vi "MGI Running Average(DBL[][]).vi"(5 "Averaging Size":i32, 6 "Average Type(FIR)":T1, 7 "Initialize? (F)":bool, 11 "Value[chan][samp]":dbl[][](array[numeric])) -> (3 "Average[chan]":dbl[](array[numeric]))   [LabVIEW 2016]
doc: "Keep running averages of each of the input values. Infinite Impulse Response requires less processing, but it takes infinite time to arrive at a steady state value. Finite Impulse Reponse maintains an array of the specified size but is able to output means.\nThis VI is a reentrant functional global.\n\nAuthored by Shawn Walpole\nsupport@mooregoodideas.com\nwww.mooregoodideas.com\n\nCopyright (c) 2010, Moore Good Ideas, Inc.\n\nAll rights reserved.\n\nRedistribution and use in source and binary forms, with or without modification, are permitted provided that the following conditions are met:\n\n * Redistributions of source code must retain the above copyright notice, this list of conditions and the following disclaimer.\n * Redistributions in binary form must reproduce the above copyright notice, this list of conditions and the following disclaimer in the documentation and/or other materials provided with the distribution.\n * Neither the name of Moore Good Ideas, Inc. nor the names of its contributors may be used to endorse or promote products derived from this software without specific prior written permission.\n\nTHIS SOFTWARE IS PROVIDED BY THE COPYRIGHT HOLDERS AND CONTRIBUTORS \"AS IS\" AND ANY EXPRESS OR IMPLIED WARRANTIES, INCLUDING, BUT NOT LIMITED TO, THE IMPLIED WARRANTIES OF MERCHANTABILITY AND FITNESS FOR A PARTICULAR PURPOSE ARE DISCLAIMED. IN NO EVENT SHALL THE COPYRIGHT OWNER OR CONTRIBUTORS BE LIABLE FOR ANY DIRECT, INDIRECT, INCIDENTAL, SPECIAL, EXEMPLARY, OR CONSEQUENTIAL DAMAGES (INCLUDING, BUT NOT LIMITED TO, PROCUREMENT OF SUBSTITUTE GOODS OR SERVICES; LOSS OF USE, DATA, OR PROFITS; OR BUSINESS INTERRUPTION) HOWEVER CAUSED AND ON ANY THEORY OF LIABILITY, WHETHER IN CONTRACT, STRICT LIABILITY, OR TORT (INCLUDING NEGLIGENCE OR OTHERWISE) ARISING IN ANY WAY OUT OF THE USE OF THIS SOFTWARE, EVEN IF ADVISED OF THE POSSIBILITY OF SUCH DAMAGE."
uses:
  <userlib>/_MGI/1D Array/MGI Average Type Enum.ctl
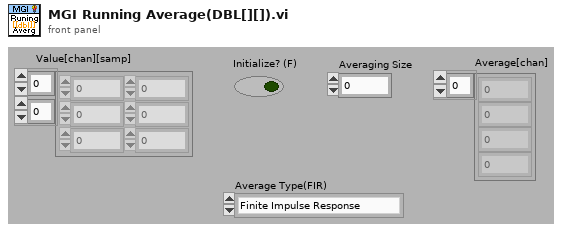
[diagram p1: front panel]
types:
  T1 = typedef "MGI Average Type Enum.ctl" = enum16{"Finite Impulse Response", "Infinite Impulse Response"}
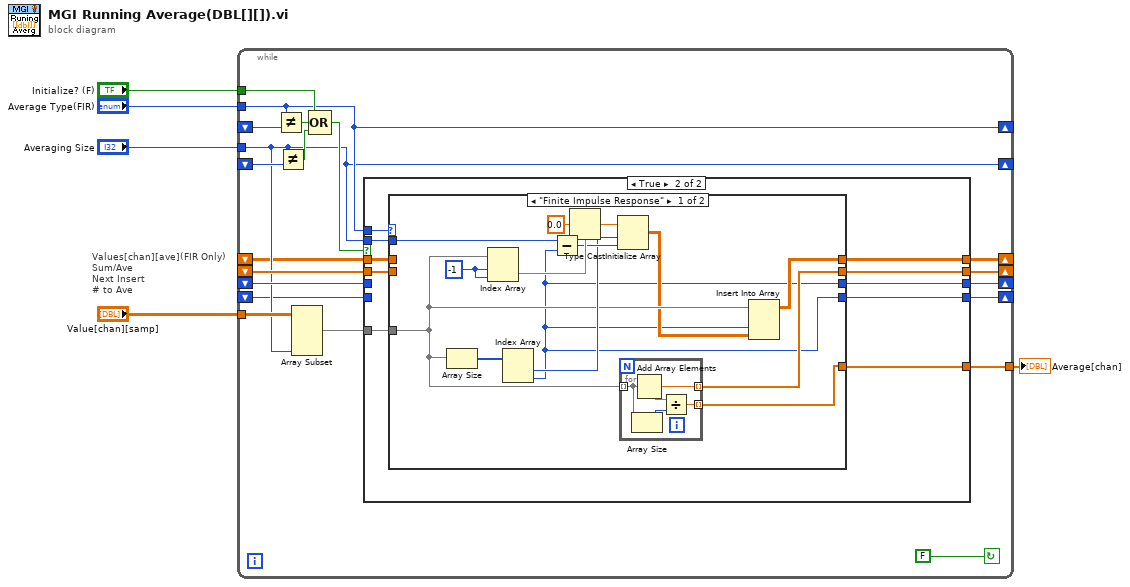
[diagram p0: block diagram]
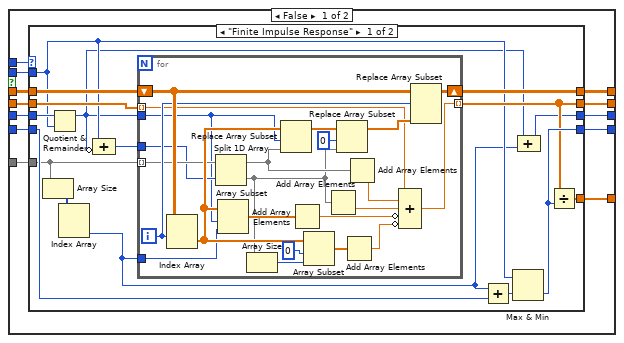
[diagram p2: hidden frame]
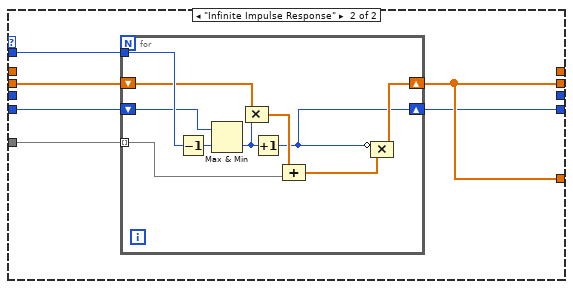
[diagram p3: hidden frame]
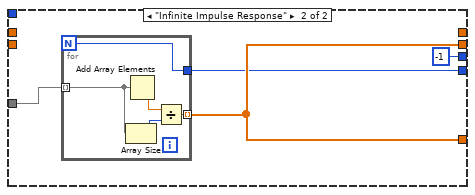
[diagram p4: hidden frame]
diagram:
  # "Values[chan][ave](FIR Only)\nSum/Ave\nNext Insert\n# to Ave"
  n1 = while {
    tunnel: "Averaging Size" -> [w9]
    tunnel: "Value[chan][samp]" -> [w11]
    shift-left: _ -> [w18]
    shift-right: [w20] -> _
    tunnel: "Initialize? (F)" -> [w23]
    shift-left: _ -> [w6]
    shift-right: [w17] -> _
    tunnel: "Average Type(FIR)" -> [w15]
    shift-right: [w15] -> _
    shift-left: _ -> [w24]
    shift-right: [w21] -> _
    shift-left: _ -> [w19]
    shift-right: [w9] -> _
    shift-left: _ -> [w22]
    tunnel: [w16] -> w2
    shift-right: [w8] -> _
    shift-left: _ -> [w7]
    stop <- FALSE continue-if-true
    n2 = Not Equal?(x=w15, y=w24) -> (x != y?=w14:bool)
    n3 = Not Equal?(x=w9, y=w22) -> (x != y?=w12:bool)
    n4 = Array Subset(array=w11, length (col)=w9) -> (w10:dbl[][])  [unwired: 3 in]
    n5 = Compound Arithmetic op=OR(w23, w14, w12) -> (w13:bool)
    n6 = case shown="True" w13 {
      tunnel: [w31 w94] -> w21
      tunnel: w10 -> [w33 w97]
      tunnel: [w29 w96] -> w20
      tunnel: w19 -> [w36 _]
      tunnel: w18 -> [w35 w100]
      tunnel: w6 -> [w34 w98]
      tunnel: w9 -> [w32 w101]
      tunnel: w15 -> [w37 w102]
      tunnel: [w30 w99] -> w17
      tunnel: [w28 w95] -> w16
      tunnel: [w26 w93] -> w8
      tunnel: w7 -> [w27 _]
      frame False {
        n7 = case shown="\"Finite Impulse Response\"" w37 {
          tunnel: w36 -> [w43 _]
          tunnel: w35 -> [w52 w81]
          tunnel: w34 -> [w53 _]
          tunnel: w33 -> [w45 w80]
          tunnel: w32 -> [w42 w82]
          tunnel: [w39 _] -> w31
          tunnel: [w51 _] -> w30
          tunnel: [w47 w78] -> w29
          tunnel: [w50 w78] -> w28
          tunnel: w27 -> [w46 w79]
          tunnel: [w48 w77] -> w26
          frame "Finite Impulse Response" {
            n8 = Array Size(array=w45) -> (size(s)=w44:i32[])
            n9 = Quotient & Remainder(x=w43, y=w42) -> (x-y*floor(x/y)=w40:i32)  [unwired: 1 out]
            n10 = Index Array(array=w44) -> (element #2=w38:i32)  [unwired: 2 in, 1 out]
            n11 = Compound Arithmetic op=ADD(w42, invert w40) -> (w41:i32)
            n12 = for {
              tunnel: w45 -> [w61] mode=indexing
              shift-right: [w75] -> w51
              shift-left: w53 -> [w76]
              tunnel: w52 -> [w70] mode=indexing
              tunnel: [w68] -> w47 mode=indexing
              tunnel: w38 -> [w54]
              tunnel: w41 -> [w60]
              tunnel: w40 -> [w55]
              i -> [w74]
              n13 = Index Array(array=w76, index (row)=w74) -> (element=w73:dbl[])  [unwired: 1 in]
              n14 = Split 1D Array(array=w61, index=w60) -> (first subarray=w59:dbl[], second subarray=w57:dbl[])
              n15 = Array Subset(array=w73, index=w55, length=w54) -> (w67:dbl[])
              n16 = Array Size(array=w57) -> (size(s)=w56:i32)
              n17 = Replace Array Subset(array=w73, new element=w59, index=w55) -> (w72:dbl[])
              n18 = Add Array Elements(numeric array=w67) -> (sum=w66:dbl)
              n19 = Array Subset(array=w73, index=0, length=w56) -> (w69:dbl[])
              n20 = Add Array Elements(numeric array=w57) -> (sum=w64:dbl)
              n21 = Replace Array Subset(array=w72, new element=w57, index=0) -> (w71:dbl[])
              n22 = Add Array Elements(numeric array=w69) -> (sum=w65:dbl)
              n23 = Add Array Elements(numeric array=w59) -> (sum=w63:dbl)
              n24 = Compound Arithmetic op=ADD(w70, w63, w64, invert w66, invert w65) -> (w68:dbl)
              n25 = Replace Array Subset(array=w76, new element=w71, index (row)=w74) -> (w75:dbl[][])  [unwired: 1 in]
            }
            n26 = Add(x=w38, y=w46) -> (x+y=w49:i32)
            n27 = Max & Min(x=w42, y=w49) -> (min(x,y)=w48:i32)  [unwired: 1 out]
            n28 = Compound Arithmetic op=ADD(w40, w38) -> (w39:i32)
            n29 = Divide(x=w47, y=w48) -> (x/y=w50:dbl[])
          }
          frame "Infinite Impulse Response" {
            n30 = for {
              tunnel: w82 -> [w92]
              tunnel: w80 -> [w89] mode=indexing
              shift-right: [w85] -> w78
              shift-left: w81 -> [w90]
              shift-right: [w83] -> w77
              shift-left: w79 -> [w84]
              n31 = Decrement(x=w92) -> (x-1=w91:i32)
              n32 = Max & Min(x=w84, y=w91) -> (min(x,y)=w86:i32)  [unwired: 1 out]
              n33 = Compound Arithmetic op=MULTIPLY(w90, w86) -> (w88:dbl[])
              n34 = Increment(x=w86) -> (x+1=w83:i32)
              n35 = Compound Arithmetic op=ADD(w88, w89) -> (w87:dbl[])
              n36 = Compound Arithmetic op=MULTIPLY(invert w83, w87) -> (w85:dbl[])
            }
          }
        }
      }
      frame True {
        n37 = case shown="\"Finite Impulse Response\"" w102 {
          tunnel: w101 -> [w111 _]
          tunnel: w100 -> [_ _]
          tunnel: [w105 _] -> w99
          tunnel: w98 -> [_ _]
          tunnel: w97 -> [w106 w123]
          tunnel: [w110 w124] -> w96
          tunnel: [w109 w124] -> w95
          tunnel: [w103 -1] -> w94
          tunnel: [w103 w121] -> w93
          frame "Finite Impulse Response" {
            w115 = -1 ("index (row)")
            n38 = Array Size(array=w106) -> (size(s)=w112:i32[])
            n39 = Index Array(array=w106, index (row)=w115, index (col)=w115) -> (element=w114:dbl)
            n40 = Index Array(array=w112) -> (element #1=w107:i32, element #2=w103:i32)  [unwired: 2 in]
            n41 = Subtract(x=w111, y=w103) -> (x-y=w108:i32)
            n42 = Type Cast(type=w114, x=0.0 ("element")) -> (*(type *) &x=w113:dbl)
            n43 = Initialize Array(w113, w107, w108) -> (w104:dbl[][])
            n44 = for {
              tunnel: w106 -> [w119] mode=indexing
              tunnel: [w120] -> w110 mode=indexing
              tunnel: [w117] -> w109 mode=indexing
              n45 = Array Size(array=w119) -> (size(s)=w118:i32)
              n46 = Add Array Elements(numeric array=w119) -> (sum=w120:dbl)
              n47 = Divide(x=w120, y=w118) -> (x/y=w117:dbl)
            }
            n48 = Insert Into Array(array=w106, index (col)=w103, new element=w104) -> (w105:dbl[][])  [unwired: 1 in]
          }
          frame "Infinite Impulse Response" {
            n49 = for {
              N -> [w129]
              tunnel: w123 -> [w127] mode=indexing
              tunnel: [w129] -> w121
              tunnel: [w125] -> w124 mode=indexing
              n50 = Array Size(array=w127) -> (size(s)=w126:i32)
              n51 = Add Array Elements(numeric array=w127) -> (sum=w128:dbl)
              n52 = Divide(x=w128, y=w126) -> (x/y=w125:dbl)
            }
          }
        }
      }
    }
  }
  "Average[chan]" <- w2
